vi "CRYWindow Wait sData.vi"(8 "pVIRef":refnum<vi>, 10 "sData":string, 11 "sAction":string) -> (1 "sData_Out":string)   [LabVIEW 2013]
uses:
  DataView/VIEW/CRYView Global.vi
panel:
  # "VIRefOuting Waiting for sData Boolean."
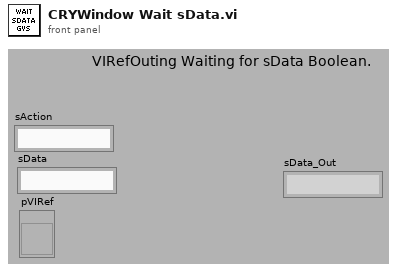
[diagram p1: front panel]
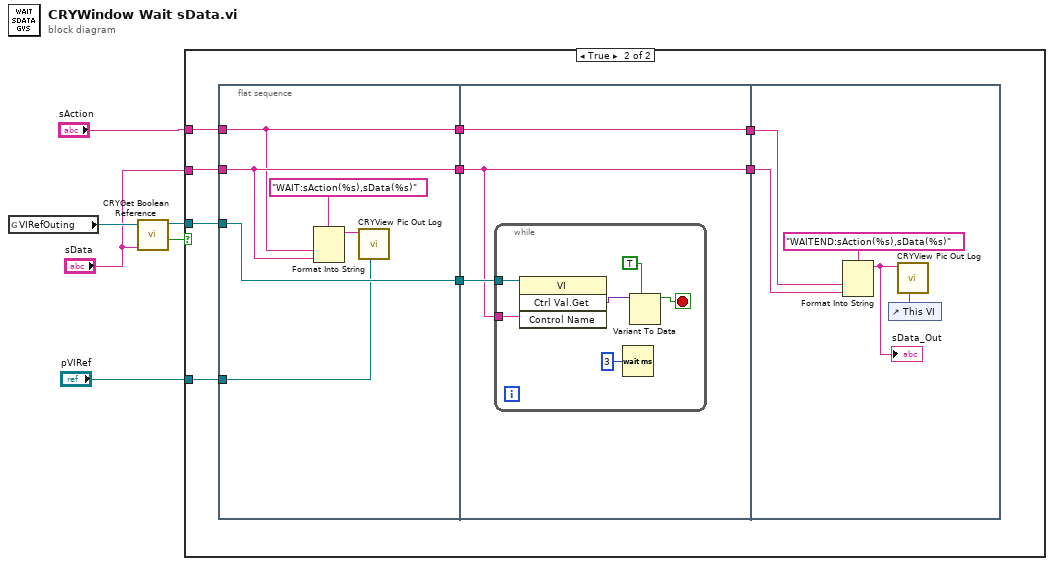
[diagram p0: block diagram]
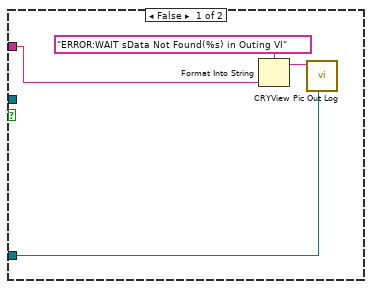
[diagram p2: hidden frame]
diagram:
  n1 = global read "CRYView Global.vi" "VIRefOuting"() -> (w5:refnum<vi>)
  n2 = call "CRYGet Boolean Reference.vi"("Label Name"="sData", "VI Refnum"=w5) -> ("Exist?"=w4:bool, "VI Refnum Out"=w6:refnum<vi>)  [unwired: 7 in, 1 out]
  n3 = case shown="True" w4 {
    tunnel: w6 -> [_ w16]
    tunnel: "pVIRef" -> [w8 w15]
    tunnel: "sData" -> [w7 w14]
    tunnel: "sAction" -> [_ w12]
    frame False {
      n4 = Format Into String(format string="ERROR:WAIT sData Not Found(%s) in Outing VI" ("string"), w7) -> (resulting string=w9:string)  [unwired: 2 in, 1 out]
      n5 = call "CRYView Pic Out Log.vi"("vi reference"=w8, "sData"=w9) -> ()  [unwired: 10 in]
    }
    frame True {
      n6 = flat-sequence {
        tunnel: w16 -> [w24]
        tunnel: w15 -> [w22]
        tunnel: [w24] -> w19
        tunnel: [w21] -> w18
        tunnel: w14 -> [w21]
        tunnel: [w20] -> w13
        tunnel: w12 -> [w20]
        tunnel: w19 -> [w28]
        tunnel: w18 -> [w27]
        tunnel: [w27] -> w17
        tunnel: w13 -> [w26]
        tunnel: [w26] -> w11
        tunnel: w17 -> [w38]
        tunnel: w11 -> [w37]
        frame #0 {
          n7 = Format Into String(format string="WAIT:sAction(%s),sData(%s)" ("string"), w20, w21) -> (resulting string=w23:string)  [unwired: 2 in, 1 out]
          n8 = call "CRYView Pic Out Log.vi"("vi reference"=w22, "sData"=w23) -> ()  [unwired: 10 in]
        }
        frame #1 {
          n9 = while {
            tunnel: w28 -> [w34]
            tunnel: w27 -> [w29]
            stop <- w31 stop-if-true
            n10 = invoke class="VI" method="Ctrl Val.Get"(reference=w34, "Control Name"=w29) -> ("Get Control Value Variant"=w33:variant)  [unwired: 2 in, 3 out]
            n11 = Wait (ms)(milliseconds to wait=u32 3) -> ()  [unwired: 1 out]
            n12 = Variant To Data(type=TRUE, Variant=w33) -> (data=w31:bool)  [unwired: 1 in, 1 out]
          }
        }
        frame #2 {
          n13 = Format Into String(format string="WAITEND:sAction(%s),sData(%s)" ("string"), w37, w38) -> (resulting string=w35:string)  [unwired: 2 in, 1 out]
          "sData_Out" <- w35
          n14 = control-ref of="This VI"() -> (w36:refnum<vi>)
          n15 = call "CRYView Pic Out Log.vi"("vi reference"=w36, "sData"=w35) -> ()  [unwired: 10 in]
        }
      }
    }
  }
